vi "MAIN_define_all_queue.vi"(8 "error in":errorcluster) -> (0 "queue ASI stage":refnum<queue>, 1 "queue CAMERA":refnum<queue>, 2 "queue DAQ":refnum<queue>, 3 "queue valve":refnum<queue>, 4 "queue piezo":refnum<queue>, 5 "queue pump":refnum<queue>, 6 "error out":errorcluster, 7 "queue FPGA":refnum<queue>, 11 "queue MAIN":refnum<queue>)   [LabVIEW 2015]
uses:
  CONTROLS/Q_camera_element.ctl
  CONTROLS/Q_main_element.ctl
  CONTROLS/Q_ASI_stage_element.ctl
  CONTROLS/Q_DAQ_element.ctl
  CONTROLS/Q_MCL_piezo_element.ctl
  CONTROLS/Q_PUMP_element.ctl
  CONTROLS/Q_VALVE_element.ctl
  CONTROLS/Q_FPGA_element.ctl
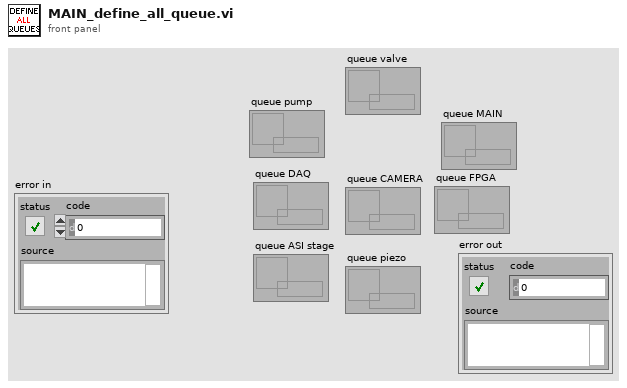
[diagram p1: front panel]
types:
  T1 = typedef "Q_FPGA_element.ctl" = cluster{"variant":variant, "Instruction":enum16{"FPGA_idle", "FPGA_initialize", "FPGA_error", "FPGA_security_stop", "FPGA_laser", "FPGA_start_stop_measure_QPD", "FPGA_measure_QPD", "FPGA_measure_QPD_noise", "FPGA_stop_measure_QPD", "FPGA_init_autofocus", "FPGA_init_single_scan", "FPGA_stop_single_scan", "FPGA_init_merFISH", "FPGA_measure_QPD_merFISH", "FPGA_init_scan_merFISH", "FPGA_scan_merFISH", "FPGA_close_merFISH", "FPGA_stop"}}
  T2 = typedef "Q_camera_element.ctl" = cluster{"variant":variant, "Instruction":enum16{"CAMERA_idle", "CAMERA_initialize", "CAMERA_error", "CAMERA_security_stop", "CAMERA_not_acquiring", "CAMERA_acquiring", "CAMERA_start_acquiring", "CAMERA_stop_acquiring", "CAMERA_change_exposure", "CAMERA_define_ROI", "CAMERA_cooler", "CAMERA_acquire_movie", "CAMERA_init_scan", "CAMERA_check_image_scan", "CAMERA_close_scan", "CAMERA_init_merFISH", "CAMERA_start_acquiring_merFISH", "CAMERA_close_scan_merFISH", "CAMERA_close_merFISH", "CAMERA_STOP"}}
  T3 = typedef "Q_VALVE_element.ctl" = cluster{"variant":variant, "Instruction":enum16{"VALVE_idle", "VALVE_initialize", "VALVE_error", "VALVE_security_stop", "VALVE_change_position", "VALVE_two_way_valves", "VALVE_init_merFISH", "VALVE_stop"}}
  T4 = typedef "Q_PUMP_element.ctl" = cluster{"variant":variant, "Instruction":enum16{"PUMP_idle", "PUMP_initialize", "PUMP_error", "PUMP_security_stop", "PUMP_read_pressure", "PUMP_change_pressure", "PUMP_init_merFISH", "PUMP_change_presure_merFISH", "PUMP_zero_pressure_merFISH", "PUMP_close_merFISH", "PUMP_stop"}}
  T5 = typedef "Q_MCL_piezo_element.ctl" = cluster{"variant":variant, "Instruction":enum16{"Piezo_idle", "Piezo_initialize", "Piezo_error", "Piezo_security_stop", "Piezo_read_z", "Piezo_move_z", "Piezo_keyboard_move", "Piezo_close_autofocus_calibration_ramp", "Piezo_change_init_state", "Piezo_init_autofocus", "Piezo_init_autofocus_merFISH_TL", "Piezo_autofocus", "Piezo_autofocus_merFISH_TL", "Piezo_stop_autofocus", "Piezo_stop_autofocus_merFISH_TL", "Piezo_autofocus_lost", "Piezo_resume_autofocus_merFISH_TL", "Piezo_check_z_position_merFISH_TL", "Piezo_init_ramp", "Piezo_move_z_ramp", "Piezo_close_ramp", "Piezo_close_merFISH", "Piezo_stop"}}
  T6 = typedef "Q_DAQ_element.ctl" = cluster{"variant":variant, "Instruction":enum16{"DAQ_idle", "DAQ_initialize", "DAQ_error", "DAQ_security_stop", "DAQ_init_single_scan", "DAQ_single_scan", "DAQ_init_merFISH", "DAQ_scan_merFISH", "DAQ_photobleaching_merFISH", "DAQ_close_merFISH", "DAQ_stop"}}
  T7 = typedef "Q_ASI_stage_element.ctl" = cluster{"variant":variant, "Instruction":enum16{"ASI_idle", "ASI_initialize", "ASI_error", "ASI_security_stop", "ASI_read_XYZ", "ASI_up", "ASI_down", "ASI_left", "ASI_right", "ASI_save_XY", "ASI_move_to_XY", "ASI_brightfield", "ASI_init_scan", "ASI_init_merFISH", "ASI_move_to_XY_merFISH", "ASI_move_to_Z_merFISH", "ASI_init_autofocus_search_merFISH", "ASI_close_autofocus_search_merFISH", "ASI_adjust_piezo_autofocus_merFISH", "ASI_set_piezo_autofocus_to_reference_position_merFISH_TL", "ASI_close_merFISH", "ASI_stop"}}
  T8 = typedef "Q_main_element.ctl" = cluster{"variant":variant, "Instruction":enum16{"Main_idle", "Main_initialize", "Main_initialize_TDMS", "Main_initialize_Queue", "Main_error", "Main_DAQ_initialization_results", "Main_ASI_initialization_results", "Main_Piezo_initialization_results", "Main_Valve_initialization_results", "Main_Pump_initialization_results", "Main_CAMERA_initialization_results", "Main_FPGA_initialization_results", "Main_DAQ_error", "Main_ASI_error", "Main_Piezo_error", "Main_CAMERA_error", "Main_Valve_error", "Main_Pump_error", "Main_FPGA_error", "Main_start_acquiring", "Main_not_acquiring", "Main_acquiring", "Main_stop_acquiring", "Main_change_exposure", "Main_change_z_scan_parameters", "Main_define_ROI", "Main_define_mosaic", "Main_read_kinetic_time", "Main_cooler", "Main_read_temperature", "Main_save_XY", "Main_load_XY", "Main_discard_XY", "Main_move_to_XY", "Main_measure_QPD", "Main_autofocus_calibration", "Main_autofocus_initialization", "Main_autofocus_stop", "Main_save_PID", "Main_change_H_valve_position", "Main_two_way_valve", "Main_save_movie", "Main_init_single_scan", "Main_single_scan", "Main_stop_single_scan", "Main_merFISH_illumination_parameters", "Main_merFISH_buffer_probe_list", "Main_merFISH_injections_procedure", "Main_merFISH_save_setpoint", "Main_merFISH_DAPI_parameters", "Main_merFISH_Brightfield_parameters", "Main_merFISH_save_embryo_ROI", "Main_merFISH_init", "Main_merFISH_resume", "Main_merFISH_start_autofocus", "Main_merFISH_open_close_valve_merFISH", "Main_merFISH_open_close_valve_photobleaching", "Main_merFISH_hybridization", "Main_merFISH_move_to_ROI", "Main_merFISH_wait_stabilization", "Main_merFISH_move_to_REF", "Main_merFISH_scan", "Main_merFISH_photobleaching_injection", "Main_merFISH_photobleaching", "Main_merFISH_send_email", "Main_merFISH_close", "Main_STOP"}}
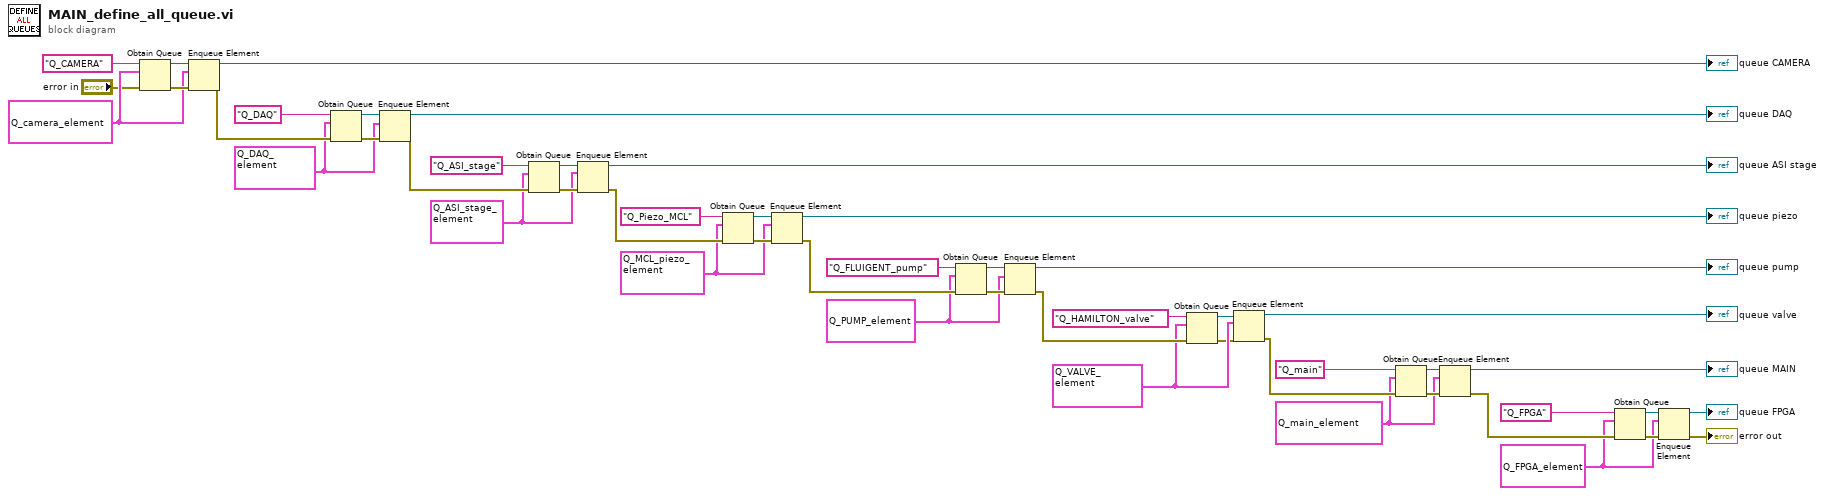
[diagram p0: block diagram]
diagram:
  w2 = T1 {"variant"=variant, "Instruction"=enum."FPGA_idle"} ("Q_VALVE")
  w15 = T2 {"variant"=variant, "Instruction"=enum."CAMERA_idle"} ("Q_ANDOR_element")
  w18 = T3 {"variant"=variant, "Instruction"=enum."VALVE_idle"} ("Q_VALVE")
  w11 = T4 {"variant"=variant, "Instruction"=enum."PUMP_idle"} ("Q_PUMP")
  w12 = T5 {"variant"=variant, "Instruction"=enum."Piezo_idle"} ("Q_MCL_Piezo")
  w14 = T6 {"variant"=variant, "Instruction"=enum."DAQ_idle"} ("Q_DAQ")
  w13 = T7 {"variant"=variant, "Instruction"=enum."ASI_idle"} ("Q_ASI_stage")
  w10 = T8 {"variant"=variant, "Instruction"=enum."Main_initialize"} ("Q_main_element")
  n1 = Obtain Queue(name (unnamed)="Q_CAMERA", element data type=w15, error in (no error)="error in") -> (queue out=w48:refnum<queue>, error out=w47:errorcluster)  [unwired: 2 in, 1 out]
  n2 = Enqueue Element(queue=w48, element=w15, error in (no error)=w47) -> (queue out=→"queue CAMERA":refnum<queue>, error out=w42:errorcluster)  [unwired: 1 in, 1 out]
  n3 = Obtain Queue(name (unnamed)="Q_DAQ", element data type=w14, error in (no error)=w42) -> (queue out=w44:refnum<queue>, error out=w45:errorcluster)  [unwired: 2 in, 1 out]
  n4 = Enqueue Element(queue=w44, element=w14, error in (no error)=w45) -> (queue out=→"queue DAQ":refnum<queue>, error out=w34:errorcluster)  [unwired: 1 in, 1 out]
  n5 = Obtain Queue(name (unnamed)="Q_ASI_stage", element data type=w13, error in (no error)=w34) -> (queue out=w36:refnum<queue>, error out=w35:errorcluster)  [unwired: 2 in, 1 out]
  n6 = Enqueue Element(queue=w36, element=w13, error in (no error)=w35) -> (queue out=→"queue ASI stage":refnum<queue>, error out=w29:errorcluster)  [unwired: 1 in, 1 out]
  n7 = Obtain Queue(name (unnamed)="Q_Piezo_MCL", element data type=w12, error in (no error)=w29) -> (queue out=w28:refnum<queue>, error out=w31:errorcluster)  [unwired: 2 in, 1 out]
  n8 = Enqueue Element(queue=w28, element=w12, error in (no error)=w31) -> (queue out=→"queue piezo":refnum<queue>, error out=w25:errorcluster)  [unwired: 1 in, 1 out]
  n9 = Obtain Queue(name (unnamed)="Q_FLUIGENT_pump", element data type=w11, error in (no error)=w25) -> (queue out=w23:refnum<queue>, error out=w26:errorcluster)  [unwired: 2 in, 1 out]
  n10 = Enqueue Element(queue=w23, element=w11, error in (no error)=w26) -> (queue out=→"queue pump":refnum<queue>, error out=w20:errorcluster)  [unwired: 1 in, 1 out]
  n11 = Obtain Queue(name (unnamed)="Q_HAMILTON_valve", element data type=w18, error in (no error)=w20) -> (queue out=w19:refnum<queue>, error out=w16:errorcluster)  [unwired: 2 in, 1 out]
  n12 = Enqueue Element(queue=w19, element=w18, error in (no error)=w16) -> (queue out=→"queue valve":refnum<queue>, error out=w17:errorcluster)  [unwired: 1 in, 1 out]
  n13 = Obtain Queue(name (unnamed)="Q_main", element data type=w10, error in (no error)=w17) -> (queue out=w40:refnum<queue>, error out=w41:errorcluster)  [unwired: 2 in, 1 out]
  n14 = Enqueue Element(queue=w40, element=w10, error in (no error)=w41) -> (queue out=→"queue MAIN":refnum<queue>, error out=w4:errorcluster)  [unwired: 1 in, 1 out]
  n15 = Obtain Queue(name (unnamed)="Q_FPGA", element data type=w2, error in (no error)=w4) -> (queue out=w6:refnum<queue>, error out=w5:errorcluster)  [unwired: 2 in, 1 out]
  n16 = Enqueue Element(queue=w6, element=w2, error in (no error)=w5) -> (queue out=→"queue FPGA":refnum<queue>, error out=→"error out":errorcluster)  [unwired: 1 in, 1 out]
